vi "Get Slave Device Info.vi"(0 "System no.":i32=1, 5 "error in":errorcluster) -> (14 "Slave Device Info":cluster{"Slave ID":i32, "*IDN? Answer":string}[](array[cluster]), 19 "error out":errorcluster)   [LabVIEW 2026]
doc: "This VI queries VER? and lists all connected DaisyChain slave devices."
uses:
  <vilib>/regexp/Match Regular Expression.xnode
panel:
  # "This VI queries VER? and lists all connected DaisyChain slave devices."
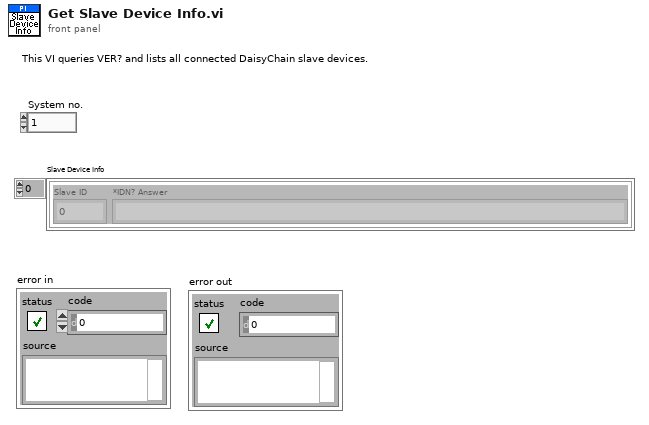
[diagram p1: front panel]
types:
  T1 = cluster{"Slave ID":i32, "après la correspondance":string}[]
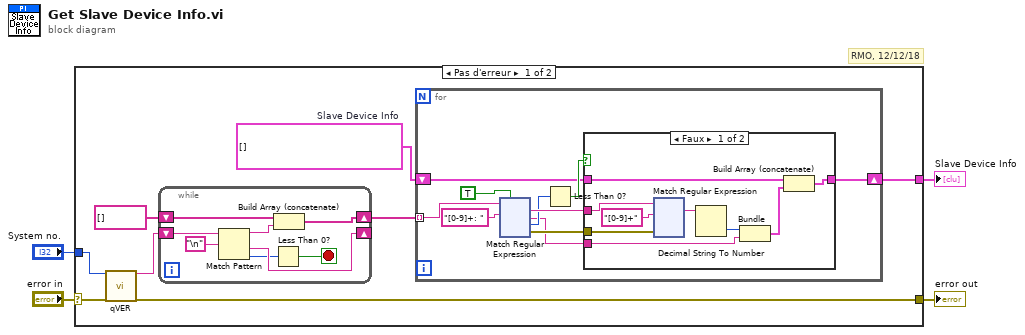
[diagram p0: block diagram]
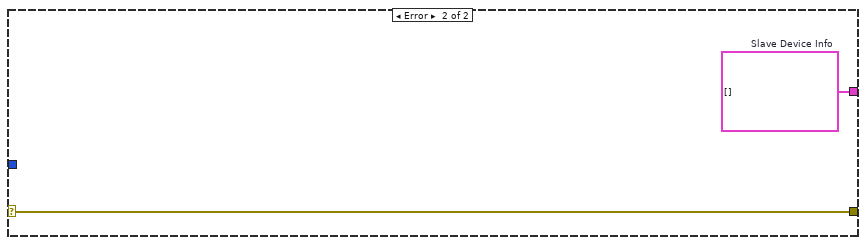
[diagram p3: hidden frame]
diagram:
  # "RMO, 12/12/18"
  n1 = case shown="Pas d'erreur" "error in" {
    selector: "error in" -> [w5 w276]
    tunnel: [w12 w275] -> w4
    tunnel: [w8 w276] -> w3
    tunnel: "System no." -> [w6 _]
    frame No Error {
      w11 = cluster{"Slave ID":i32, "*IDN? Answer":string}[] []  # Slave Device Info
      n2 = call "qVER.vi"("System no."=w6, "error in"=w5) -> ("Firmware version"=w10:string, "error out"=w8:errorcluster)  [unwired: 16 out]
      n3 = while {
        shift-right: [w270] -> _
        shift-left: w10 -> [w274]
        shift-right: [w269] -> w9
        shift-left: string[] [] -> [w272]
        stop <- w267 stop-if-true
        n4 = Match Pattern(string=w274, regular expression="\n") -> (before substring=w271:string, after substring=w270:string, offset past match=w268:i32)  [unwired: 2 out]
        n5 = Less Than 0?(x=w268) -> (x < 0?=w267:bool)
        n6 = Build Array (concatenate)(w272, w271) -> (w269:string[])
      }
      n7 = for {
        tunnel: w9 -> [w22] mode=indexing
        shift-right: [w13] -> w12
        shift-left: w11 -> [w14]
        n8 = xnode "Match Regular Expression"("chaîne en entrée"=w22, "expression régulière"="[0-9]+: " ("regular expression"), "ignorer la casse ? (F)"=TRUE) -> ("toute l'expression"=w18:string, "après la correspondance"=w15:string, "offset après correspondance"=w17:i32, "sortie d'erreur"=w19:errorcluster)  [unwired: 2 in, 2 out]
        n9 = Less Than 0?(x=w17) -> (x < 0?=w16:bool)
        n10 = case shown="Faux" w16 {
          tunnel: w19 -> [w31 _]
          tunnel: w18 -> [w30 _]
          tunnel: w15 -> [w26 _]
          tunnel: w14 -> [w24 w149]
          tunnel: [w23 w149] -> w13
          frame False {
            n11 = xnode "Match Regular Expression"("chaîne en entrée"=w30, "expression régulière"="[0-9]+" ("regular expression"), "entrée d'erreur"=w31) -> ("toute l'expression"=w28:string)  [unwired: 1 in, 6 out]
            n12 = Decimal String To Number(string=w28) -> (number=w27:i32)  [unwired: 3 out]
            n13 = Bundle(w27, "après la correspondance"=w26) -> (w25:cluster{i32, "après la correspondance":string})  [unwired: 1 out]
            n14 = Build Array (concatenate)(w24, w25) -> (w23:T1)
          }
          frame True {
          }
        }
      }
    }
    frame Error {
      w275 = cluster{"Slave ID":i32, "*IDN? Answer":string}[] []  # Slave Device Info
    }
  }
  "Slave Device Info" <- w4
  "error out" <- w3
